vi "A Test history.vi"(8 "错误输入（无错误）":errorcluster, 10 "Fitted Circle (Find Circular Edge 1)":T1 {"Average SNR (dB)" format="%.2f"; "Average Strength" format="%.2f"; "Roundness (Real-World)" format="%.2f"; "Radius (Real-World)" format="%.2f"; "Center (Real-World)"."Y" format="%.2f"; "Center (Real-World)"."X" format="%.2f"; "Radius (Pixels)" format="%.2f"; "Center (Pixels)"."Y" format="%.2f"; "Center (Pixels)"."X" format="%.2f"}, 11 "Tbl引用句柄":refnum<vi>) -> (0 "错误输出":errorcluster, 3 "F-格式字符串":string)   [LabVIEW 2017]
uses:
  Global System.vi
panel:
  out "x+y":dbl
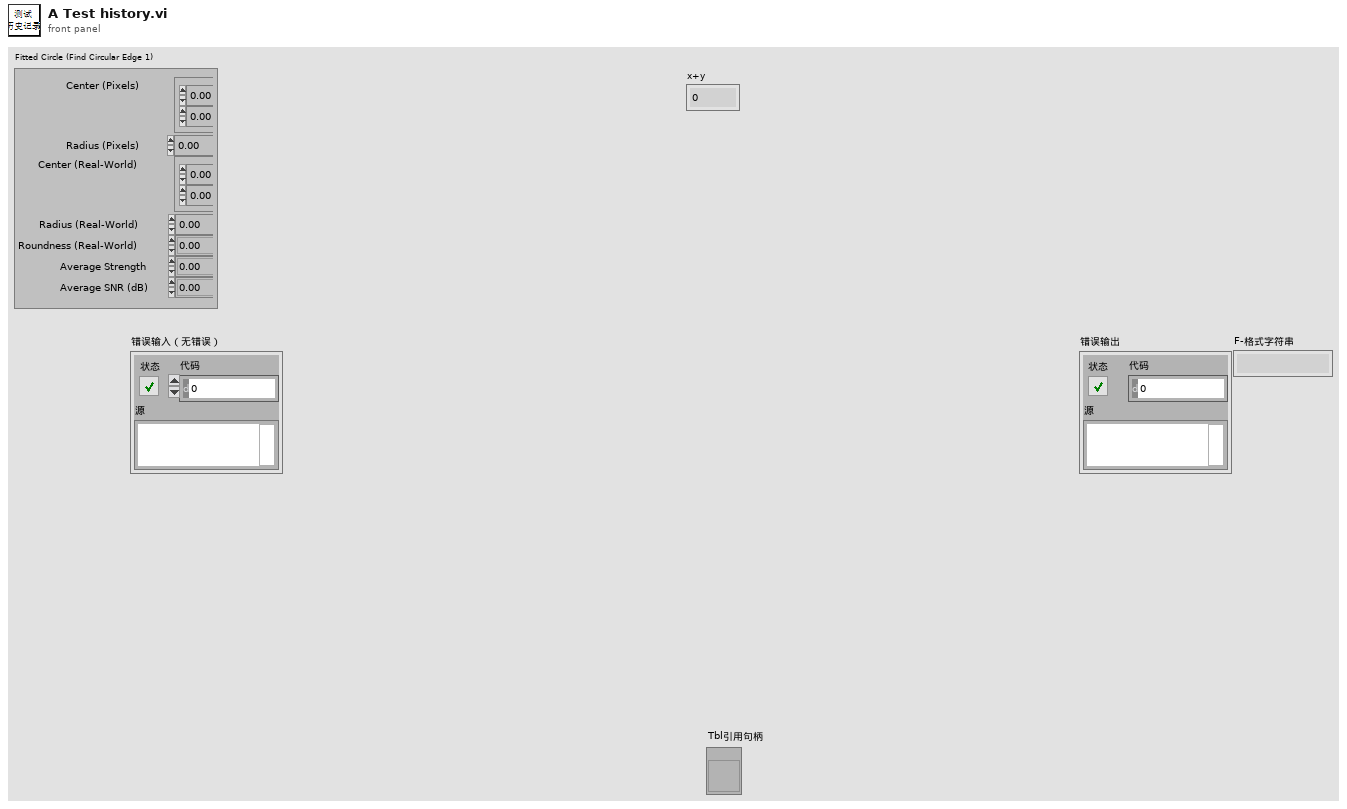
[diagram p1: front panel]
types:
  T1 = cluster{"Center (Pixels)":cluster{"X":sgl, "Y":sgl}, "Radius (Pixels)":dbl, "Center (Real-World)":cluster{"X":sgl, "Y":sgl}, "Radius (Real-World)":dbl, "Roundness (Real-World)":dbl, "Average Strength":dbl, "Average SNR (dB)":dbl}
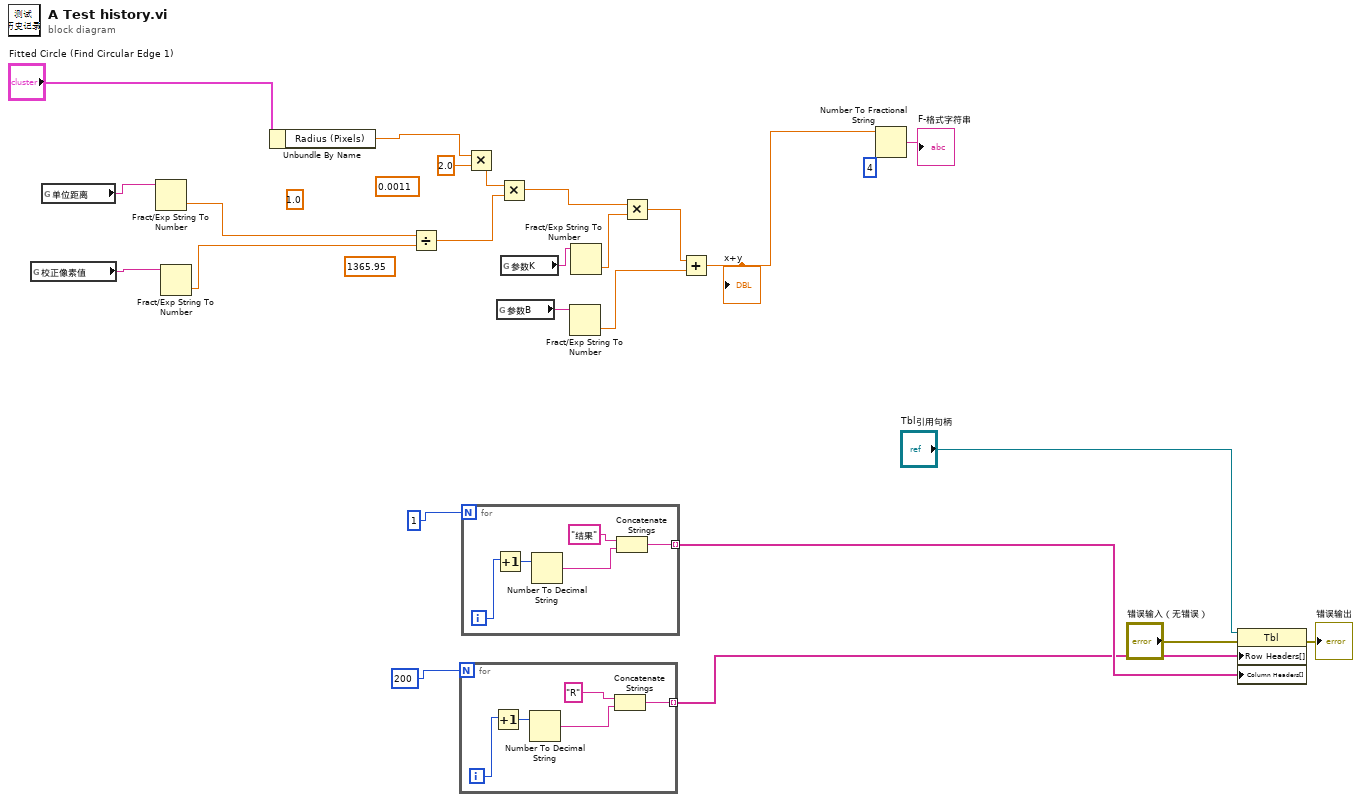
[diagram p0: block diagram]
diagram:
  (unwired) 1365.95 ("y")
  (unwired) 1.0 ("x")
  (unwired) 0.0011 ("y")
  n1 = global read "Global System.vi" "校正像素值"() -> (w9:string)
  n2 = global read "Global System.vi" "单位距离"() -> (w11:string)
  n3 = Fract/Exp String To Number(string=w11) -> (number=w10:dbl)  [unwired: 3 in, 1 out]
  n4 = Fract/Exp String To Number(string=w9) -> (number=w8:dbl)  [unwired: 3 in, 1 out]
  n5 = Unbundle By Name("Fitted Circle (Find Circular Edge 1)") -> ("Radius (Pixels)"=w14:dbl)
  n6 = Divide(x=w10, y=w8) -> (x/y=w12:dbl)
  n7 = for {
    N: 200 -> [_]
    tunnel: [w28] -> w21 mode=indexing
    i -> [w27]
    n8 = Increment(x=w27) -> (x+1=w26:i32)
    n9 = Number To Decimal String(number=w26) -> (decimal integer string=w29:string)  [unwired: 1 in]
    n10 = Concatenate Strings("R", w29) -> (w28:string)
  }
  n11 = for {
    N: 1 -> [_]
    tunnel: [w33] -> w23 mode=indexing
    i -> [w32]
    n12 = Increment(x=w32) -> (x+1=w31:i32)
    n13 = Number To Decimal String(number=w31) -> (decimal integer string=w34:string)  [unwired: 1 in]
    n14 = Concatenate Strings("结果", w34) -> (w33:string)
  }
  n15 = Multiply(x=w14, y=2.0) -> (x*y=w15:dbl)
  n16 = global read "Global System.vi" "参数B"() -> (w6:string)
  n17 = Multiply(x=w15, y=w12) -> (x*y=w2:dbl)
  n18 = global read "Global System.vi" "参数K"() -> (w7:string)
  n19 = Fract/Exp String To Number(string=w6) -> (number=w3:dbl)  [unwired: 3 in, 1 out]
  n20 = Fract/Exp String To Number(string=w7) -> (number=w5:dbl)  [unwired: 3 in, 1 out]
  n21 = Multiply(x=w2, y=w5) -> (x*y=w4:dbl)
  n22 = Add(x=w4, y=w3) -> (x+y=w1:dbl)
  "x+y" <- w1
  n23 = Number To Fractional String(number=w1, precision (6)=i16 4 ("精度(6)")) -> (F-format string=→"F-格式字符串":string)  [unwired: 2 in]
  n24 = property class="Tbl"(reference="Tbl引用句柄", error in="错误输入（无错误）", "Row Headers[]"=w21, "Column Headers[]"=w23) -> (error out=→"错误输出":errorcluster)  [unwired: 1 out]
